vi "Rerun Aync VI.vi"(11 "Test Case In":refnum<class "Tests Event MessengerM.lvclass">) -> (0 "error out":errorcluster, 3 "Test Case Out":refnum<class "Tests Event MessengerM.lvclass">)   [LabVIEW 2020, in "Tests Event MessengerM.lvclass"]
uses:
  Tests Event MessengerM.lvclass
  C:/Program Files/National Instruments/LabVIEW 2026/vi.lib/Astemes/LUnit/Test Case.lvclass
  <vilib>/Astemes/LUnit/Test Case.lvclass/Test Case.ctl
  <vilib>/Astemes/LUnit/Test Case.lvclass
  b79f69fd-ac2f-4806-84b0-9e56e719c1a6.vi
  ca4d2565-46c2-4d99-81da-89eaa5d06671.vi
  00c4da50-6fd3-4adb-ad10-1b482b76ad5f.vi
  ab97bdfb-d86c-4efd-8a21-5b3b2d2bdc58.vi
panel:
  in  "Stop":bool
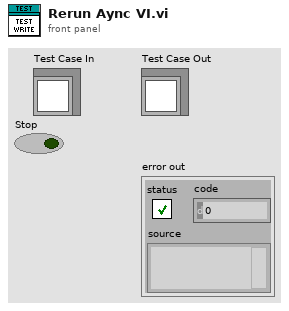
[diagram p1: front panel]
types:
  T1 = typedef "Event MessengerM-i32.lvlib/))Channel.ctl" = refnum<queue>
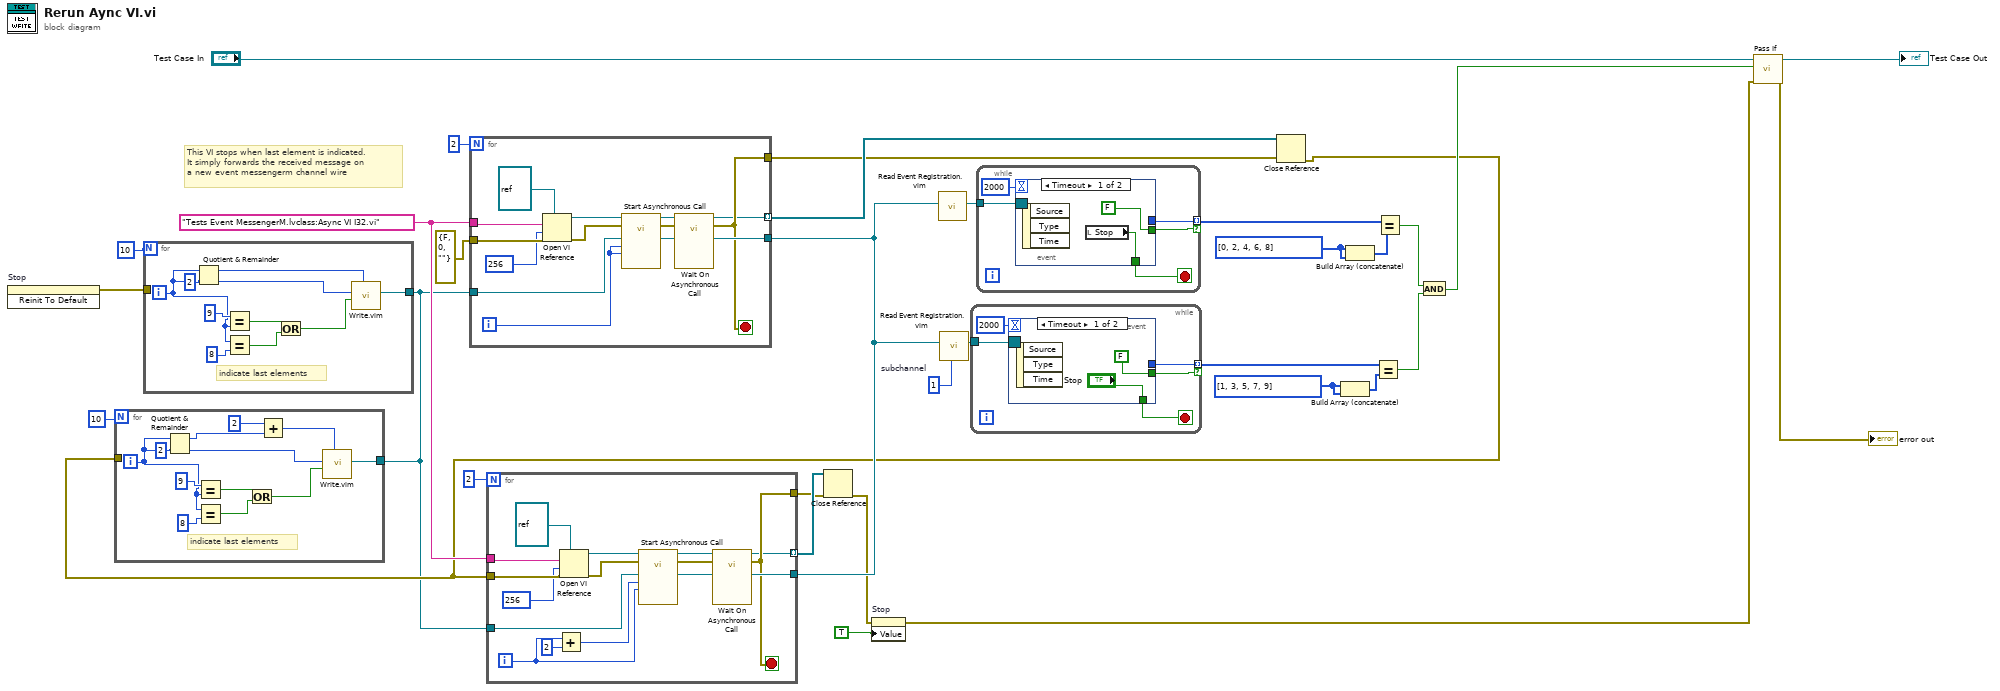
[diagram p0: block diagram]
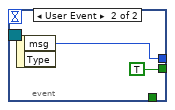
[diagram p2: hidden frame]
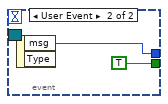
[diagram p3: hidden frame]
diagram:
  w17 = 1  # subchannel
  w16 = "Tests Event MessengerM.lvclass:Async VI I32.vi"
  w5 = i32[] [0, 2, 4, 6, 8] ("Array")
  w4 = i32[] [1, 3, 5, 7, 9] ("Array 2")
  # "This VI stops when last element is indicated.\nIt simply forwards the received message on\na new event messengerm channel wire"
  n1 = invoke on="Stop" class="Bool (strict)" method="Reinit To Default"() -> (error out=w14:errorcluster)  [unwired: 3 in, 2 out]
  n2 = Build Array (concatenate)(w4, w4) -> (w7:i32[])
  n3 = Build Array (concatenate)(w5, w5) -> (w6:i32[])
  n4 = for {
    N: 10 -> [_]
    tunnel: [w37] -> w9
    tunnel: w10 -> [_]
    i -> [w38]
    # "indicate last elements"
    n5 = Quotient & Remainder(x=w38, y=2) -> (x-y*floor(x/y)=w36:i32)  [unwired: 1 out]
    n6 = Equal?(x=9, y=w38) -> (x = y?=w41:bool)
    n7 = Equal?(x=w38, y=8 ("x")) -> (x = y?=w39:bool)
    n8 = Or(x=w41, y=w39) -> (x .or. y?=w33:bool)
    n9 = Add(x=2, y=w36) -> (x+y=w34:i32)
    n10 = call "Write.vim"("subchannel"=w34, "last message? (F)"=w33, "element"=w38) -> ("channel"=w37:T1)  [unwired: 7 in, 1 out]
  }
  n11 = for {
    N: 10 -> [_]
    tunnel: w9 -> [w46]
    tunnel: w14 -> [_]
    i -> [w47]
    # "indicate last elements"
    n12 = Quotient & Remainder(x=w47, y=2) -> (x-y*floor(x/y)=w45:i32)  [unwired: 1 out]
    n13 = Equal?(x=9, y=w47) -> (x = y?=w50:bool)
    n14 = Equal?(x=w47, y=8 ("x")) -> (x = y?=w48:bool)
    n15 = Or(x=w50, y=w48) -> (x .or. y?=w44:bool)
    n16 = call "Write.vim"("subchannel"=w45, "last message? (F)"=w44, "element"=w47) -> ("channel"=w46:T1)  [unwired: 7 in, 1 out]
  }
  n17 = for {
    N: 2 -> [_]
    tunnel: w16 -> [w65]
    tunnel: errorcluster {"status"=FALSE, "code"=0, "source"=""} ("error constant") -> [w61]
    tunnel: [w60] -> w15
    tunnel: [w54] -> w21 mode=indexing
    tunnel: [w56] -> w20
    tunnel: w9 -> [w57]
    i -> [w53]
    stop <- w56 stop-if-true
    n18 = Open VI Reference(type specifier VI Refnum (for type only)=refnum<vi> refnum, vi path=w65, options=256, error in (no error)=w61) -> (vi reference=w63:refnum<vi>, error out=w62:errorcluster)  [unwired: 2 in]
    n19 = call-by-ref "Start Asynchronous Call"(reference=w63, error in=w62, "subchannel another channel (0)"=w53, "subchannel (0)"=w53, "channel"=w57) -> (reference out=w55:refnum<vi>, error out=w58:errorcluster, "another channel"=w60:T1)  [unwired: 8 in]
    n20 = call-by-ref "Wait On Asynchronous Call"(reference=w55, error in=w58) -> (reference out=w54:refnum<vi>, error out=w56:errorcluster)  [unwired: 11 in, 1 out]
  }
  n21 = call "Read Event Registration.vim"("channel"=w15) -> ("event registration refnum"=w19:refnum<event-registration>)  [unwired: 10 in]
  n22 = call "Read Event Registration.vim"("subchannel"=w17, "channel"=w15) -> ("event registration refnum"=w18:refnum<event-registration>)  [unwired: 9 in]
  n23 = while {
    tunnel: w18 -> [w70]
    tunnel: [w67] -> w28 mode=indexing if=w66
    stop <- w69 stop-if-true
    n24 = event shown="[0] Timeout" {
      selector: w70 -> [_ _]
      dyn-events: _ -> [_ _]
      timeout: 2000 -> [_ _]
      tunnel: [_ w74] -> w67
      tunnel: ["Stop" _] -> w69
      tunnel: [FALSE TRUE] -> w66
      event Timeout {
        n25 = event-data() -> ()  [unwired: 1 in, 3 out]
      }
      event User Event {
        n26 = event-data() -> ("msg"=w74:i32)  [unwired: 1 in, 1 out]
      }
    }
  }
  n27 = while {
    tunnel: w19 -> [w79]
    tunnel: [w78] -> w26 mode=indexing if=w75
    stop <- w76 stop-if-true
    n28 = event shown="[0] Timeout" {
      selector: w79 -> [_ _]
      dyn-events: _ -> [_ _]
      timeout: 2000 -> [_ _]
      tunnel: [_ w83] -> w78
      tunnel: [w81 _] -> w76
      tunnel: [FALSE TRUE] -> w75
      event Timeout {
        n29 = event-data() -> ()  [unwired: 1 in, 3 out]
        n30 = local read "Stop"() -> (w81:bool)
      }
      event User Event {
        n31 = event-data() -> ("msg"=w83:i32)  [unwired: 1 in, 1 out]
      }
    }
  }
  n32 = Close Reference(reference=w21, error in (no error)=w20) -> (error out=w10:errorcluster)
  n33 = for {
    N: 2 -> [_]
    tunnel: w16 -> [w98]
    tunnel: w10 -> [w94]
    tunnel: w15 -> [w93]
    tunnel: [w89] -> w12
    tunnel: w9 -> [w90]
    tunnel: [w87] -> w13 mode=indexing
    i -> [w84]
    stop <- w89 stop-if-true
    n34 = Add(x=w84, y=2) -> (x+y=w86:i32)
    n35 = Open VI Reference(type specifier VI Refnum (for type only)=refnum<vi> refnum, vi path=w98, options=256, error in (no error)=w94) -> (vi reference=w96:refnum<vi>, error out=w95:errorcluster)  [unwired: 2 in]
    n36 = call-by-ref "Start Asynchronous Call"(reference=w96, error in=w95, "subchannel another channel (0)"=w84, "subchannel (0)"=w86, "channel"=w90) -> (reference out=w88:refnum<vi>, error out=w91:errorcluster, "another channel"=w93:T1)  [unwired: 8 in]
    n37 = call-by-ref "Wait On Asynchronous Call"(reference=w88, error in=w91) -> (reference out=w87:refnum<vi>, error out=w89:errorcluster)  [unwired: 11 in, 1 out]
  }
  n38 = Close Reference(reference=w13, error in (no error)=w12) -> (error out=w2:errorcluster)
  n39 = property on="Stop" class="Bool (strict)"(error in=w2, "Value"=TRUE ("Stop")) -> (error out=w1:errorcluster)  [unwired: 1 in, 1 out]
  n40 = Equal?(x=w28, y=w7) -> (x = y?=w27:bool)
  n41 = Equal?(x=w26, y=w6) -> (x = y?=w25:bool)
  n42 = And(x=w25, y=w27) -> (x .and. y?=w24:bool)
  n43 = call <vilib>:"Pass If.vi"("error in (no error)"=w1, "Pass?"=w24, "LUnit Test Case In"="Test Case In") -> ("error out"=→"error out":errorcluster, "LUnit Test Case Out"=→"Test Case Out":refnum<class "Tests Event MessengerM.lvclass">)  [unwired: 7 in]
